vi "convertps-to-mm.vi"(1 "ps":dbl, 2 "Real zero":dbl) -> (0 "mm":dbl)   [LabVIEW 2018]
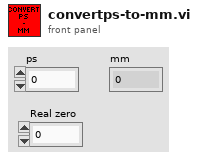
[diagram p1: front panel]
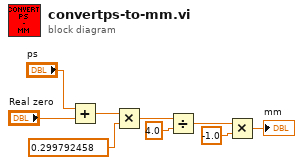
[diagram p0: block diagram]
diagram:
  n1 = Add(x="ps", y="Real zero") -> (x+y=w5:dbl)
  n2 = Multiply(x=w5, y=0.299792458) -> (x*y=w9:dbl)
  n3 = Divide(x=w9, y=4.0) -> (x/y=w3:dbl)
  n4 = Multiply(x=w3, y=-1.0) -> (x*y=→"mm":dbl)
